vi "Stepper ToGo.vi"(8 "Error In":errorcluster, 11 "ChipKit Resource":T1={"COM Port"="", "Board Type"=enum."ChipKit uC32", "Connection Type"=enum."USB / Serial", "Baud Rate (115200)"=15, "Bytes Per Packet (15)"=15}) -> (0 "Error Out":errorcluster, 1 "Steps remaining":u16, 2 "Steps Remaining?":bool, 3 "ChipKit Resource":T1={"COM Port"="", "Board Type"=enum."ChipKit uC32", "Connection Type"=enum."USB / Serial", "Baud Rate (115200)"=15, "Bytes Per Packet (15)"=15})   [LabVIEW 2011, in "LabVIEW Interface for ChipKit.lvlib"]
doc: "Check to see if the Arduino is still processing a previous step command. Wait until Steps Remaining? is false to ensure step commands aren't overwritten."
uses:
  LabVIEW Interface for ChipKit.lvlib
  Private/Type Defs/Chipkit Resource.ctl
  Private/Type Defs/Board Type.ctl
  Private/Type Defs/Connection Type.ctl
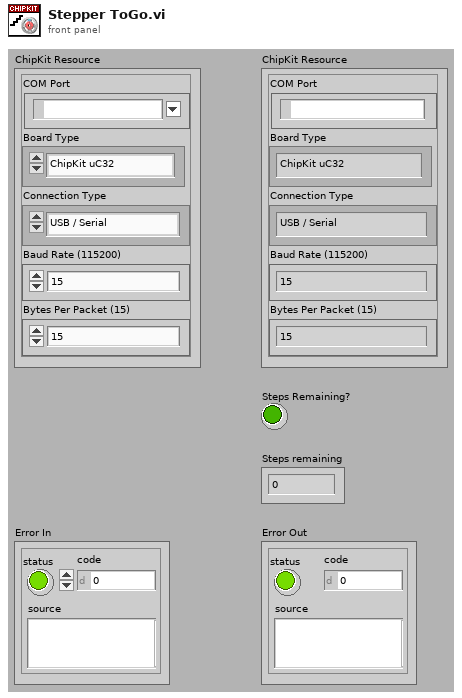
[diagram p1: front panel]
types:
  T1 = typedef "LabVIEW Interface for ChipKit.lvlib/Chipkit Resource.ctl" = cluster{"COM Port":refnum<visa-resource-name>, "Board Type":T2, "Connection Type":T3, "Baud Rate (115200)":u32, "Bytes Per Packet (15)":u32}
  T2 = typedef "LabVIEW Interface for ChipKit.lvlib/Board Type.ctl" = enum16{"ChipKit uC32", "ChipKit Uno32", "ChipKit Max32"}
  T3 = typedef "LabVIEW Interface for ChipKit.lvlib/Connection Type.ctl" = enum8{"USB / Serial", "XBEE", "BlueSmirf (Bluetooth)"}
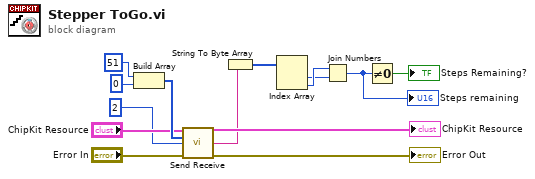
[diagram p0: block diagram]
diagram:
  n1 = Build Array(u8 51, u8 0 ("element")) -> (w7:u8[])
  n2 = call "Send Receive.vi"("Arduino Resource"="ChipKit Resource", "Data"=w7, "Bytes To Read (0)"=u8 2, "error in"="Error In") -> ("Arduino Resource"=→"ChipKit Resource":T1, "Read Buffer"=w5:string, "error out"=→"Error Out":errorcluster)  [unwired: 9 in]
  n3 = String To Byte Array(string=w5) -> (unsigned byte array=w13:u8[])
  n4 = Index Array(array=w13) -> (element #1=w10:u8, element #2=w11:u8)  [unwired: 2 in]
  n5 = Join Numbers(hi=w11, lo=w10) -> ((hi.lo)=w8:u16)
  "Steps remaining" <- w8
  n6 = Not Equal To 0?(x=w8) -> (x != 0?=→"Steps Remaining?":bool)
